vi "Insert Log.vi"(8 "error in (no error)":errorcluster caption="Error In", 9 "Data":string[][](array[string]), 10 "Table":string(combo), 11 "Project":string) -> (0 "error out":errorcluster caption="Error Out")   [LabVIEW 2020]
uses:
  006 Path Management/006 System Gloabl.vi
  <vilib>/addons/database/NI_Database_API.lvlib
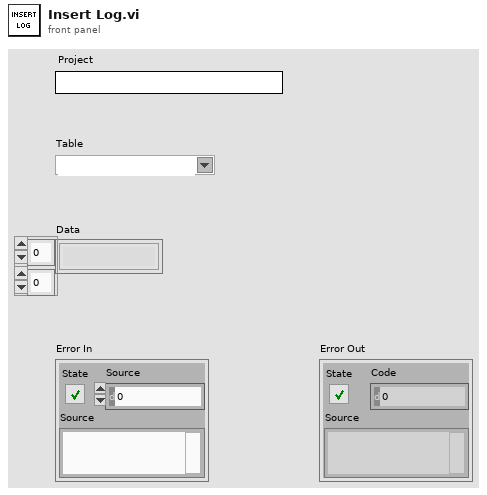
[diagram p1: front panel]
types:
  T1 = enum32{"invalid app kind", "Development System", "Run Time System", "Student Edition", "Embedded LabVIEW", "Evaluation", "Custom"}
  T2 = cluster{"Update_Time":string, "Log_Name":string, "Data_Identifier":string, "Data_Value":string}
  T3 = cluster{"Update_Time":string, "Data_Identifier":string, "Data_Operate":string, "Data_Value":string, "Warning_Level":string}
  T4 = typedef "NI_Database_API.lvlib/Conn ObjectReference.ctl" = refnum<k1>
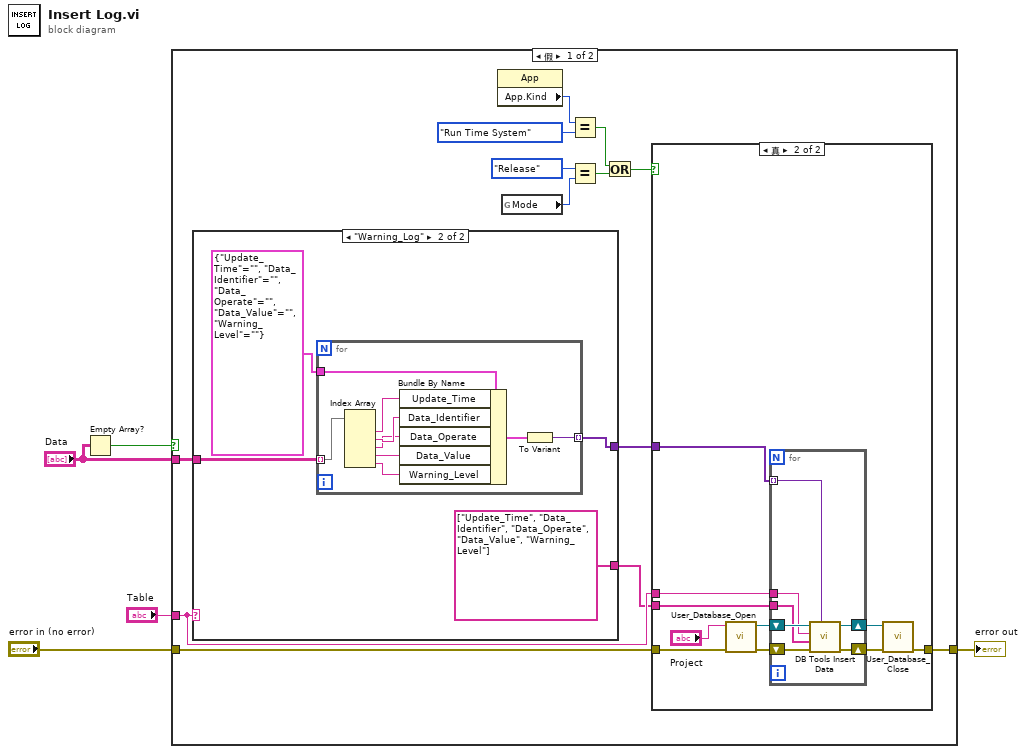
[diagram p0: block diagram]
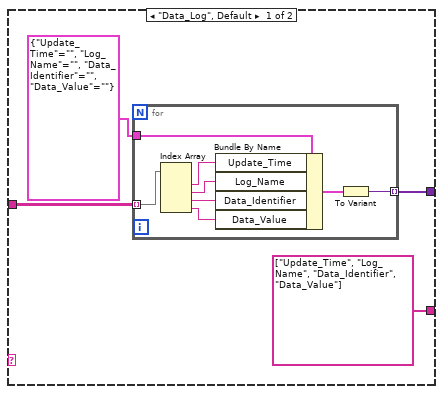
[diagram p3: hidden frame]
diagram:
  n1 = Empty Array?(array="Data") -> (empty?=w1:bool)
  n2 = case shown="假" w1 {
    tunnel: [w18 w62] -> w5
    tunnel: "Table" -> [w17 _]
    tunnel: "Data" -> [w14 _]
    tunnel: "error in (no error)" -> [w13 w62]
    frame False {
      n3 = case shown="\"Warning_Log\"" w17 {
        tunnel: [string[] ["Update_Time", "Log_Name", "Data_Identifier", "Data_Value"] string[] ["Update_Time", "Data_Identifier", "Data_Operate", "Data_Value", "Warning_Level"]] -> w16
        tunnel: [w39 w49] -> w15
        tunnel: w14 -> [w37 w51]
        frame "Data_Log", Default {
          n4 = for {
            tunnel: w37 -> [w46] mode=indexing
            tunnel: [w48] -> w39 mode=indexing
            tunnel: T2 {"Update_Time"="", "Log_Name"="", "Data_Identifier"="", "Data_Value"=""} -> [w47]
            n5 = Index Array(array=w46) -> (element #1=w45:string, element #2=w44:string, element #3=w43:string, element #4=w42:string)  [unwired: 4 in]
            n6 = Bundle By Name(cluster=w47, "Update_Time"=w45, "Log_Name"=w44, "Data_Identifier"=w43, "Data_Value"=w42) -> (w41:T2)
            n7 = To Variant(anything=w41) -> (Variant=w48:variant)
          }
        }
        frame "Warning_Log" {
          n8 = for {
            tunnel: w51 -> [w61] mode=indexing
            tunnel: T3 {"Update_Time"="", "Data_Identifier"="", "Data_Operate"="", "Data_Value"="", "Warning_Level"=""} -> [w60]
            tunnel: [w53] -> w49 mode=indexing
            n9 = Index Array(array=w61) -> (element #1=w59:string, element #2=w58:string, element #3=w57:string, element #4=w56:string, element #5=w55:string)  [unwired: 5 in]
            n10 = Bundle By Name(cluster=w60, "Update_Time"=w59, "Data_Identifier"=w58, "Data_Operate"=w57, "Data_Value"=w56, "Warning_Level"=w55) -> (w54:T3)
            n11 = To Variant(anything=w54) -> (Variant=w53:variant)
          }
        }
      }
      n12 = property class="App"() -> ("App.Kind"=w9:T1)  [unwired: 2 in, 2 out]
      n13 = global read "006 System Gloabl.vi" "Mode"() -> (w12:enum16{"Release", "Debug"})
      n14 = Equal?(x=w9, y=T1."Run Time System") -> (x = y?=w7:bool)
      n15 = Equal?(x=enum16{"Release", "Debug"}."Release", y=w12) -> (x = y?=w10:bool)
      n16 = Or(x=w7, y=w10) -> (x .or. y?=w6:bool)
      n17 = case shown="真" w6 {
        tunnel: [w19 w25] -> w18
        tunnel: w17 -> [_ w24]
        tunnel: w16 -> [_ w23]
        tunnel: w15 -> [_ w22]
        tunnel: w13 -> [w19 w21]
        frame False {
        }
        frame True {
          n18 = call "User_Database_Open.vi"("error in (no error)"=w21, "Project"="Project") -> ("error out"=w28:errorcluster, "DB Ref Out"=w29:T4)  [unwired: 8 in]
          n19 = for {
            tunnel: w24 -> [w32]
            tunnel: w23 -> [w31]
            shift-right: [w34] -> w27
            shift-left: w29 -> [w36]
            shift-right: [w33] -> w26
            shift-left: w28 -> [w35]
            tunnel: w22 -> [w30] mode=indexing
            n20 = call <vilib>:"DB Tools Insert Data.vi"("data"=w30, "error in (no error)"=w35, "columns"=w31, "table"=w32, "connection reference"=w36) -> ("error out"=w33:errorcluster, "connection reference out"=w34:T4)  [unwired: 5 in]
          }
          n21 = call "User_Database_Close.vi"("error in (no error)"=w26, "DB Ref In"=w27) -> ("error out"=w25:errorcluster)  [unwired: 9 in]
        }
      }
    }
    frame True {
    }
  }
  "error out" <- w5
